vi "_Dequeue JKISMQ.vi"(8 "Error in":errorcluster caption="Error in (no error)", 9 "Dequeue Timeout(0ms)":i32, 10 "State(s) in (\"\")":string, 11 "JKISMQ in":T1) -> (0 "Error out":errorcluster, 2 "States Out":string, 3 "JKISMQ out":T1)   [LabVIEW 2014, in "JKI State Machine++.lvlib"]
uses:
  JKI State Machine++.lvlib
  _JKISMQ.ctl
  Typedef/_Cross JKISM State Data.ctl
  Typedef/_JKISM_MSG_TYPE.ctl
  Typedef/_Cross JKISM State Response.ctl
  Typedef/_JKISM_MODE.ctl
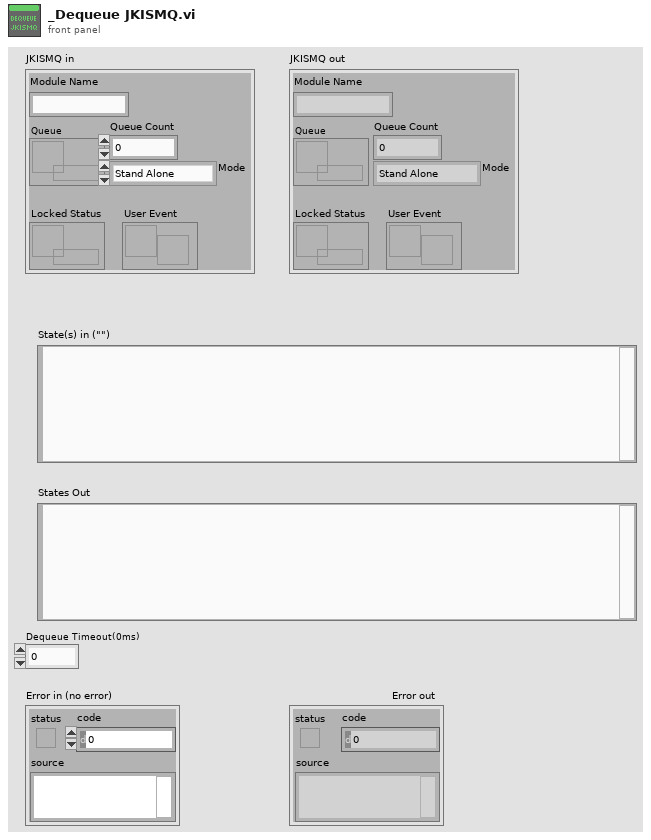
[diagram p1: front panel]
types:
  T1 = typedef "JKI State Machine++.lvlib/_JKISMQ.ctl" = cluster{"Module Name":string, "Queue":refnum<queue>, "Locked Status":refnum<data-value>, "Mode":T2, "User Event":refnum<user-event>, "Queue Count":i32}
  T2 = typedef "JKI State Machine++.lvlib/_JKISM_MODE.ctl" = enum16{"Stand Alone", "JKISM", "Action Worker"}
  T3 = typedef "JKI State Machine++.lvlib/_Cross JKISM State Data.ctl" = cluster{"Msg Type":T4, "state":string, "args":string, "source":string, "RespQ":refnum<queue>, "Pre-State":string, "Arg-State":string}
  T4 = typedef "JKI State Machine++.lvlib/_JKISM_MSG_TYPE.ctl" = enum16{"Sync Message(-@)", "Async Message(->)", "Async Response", "Broadcast(-><status>)", "Broadcast(-><interrupt>)"}
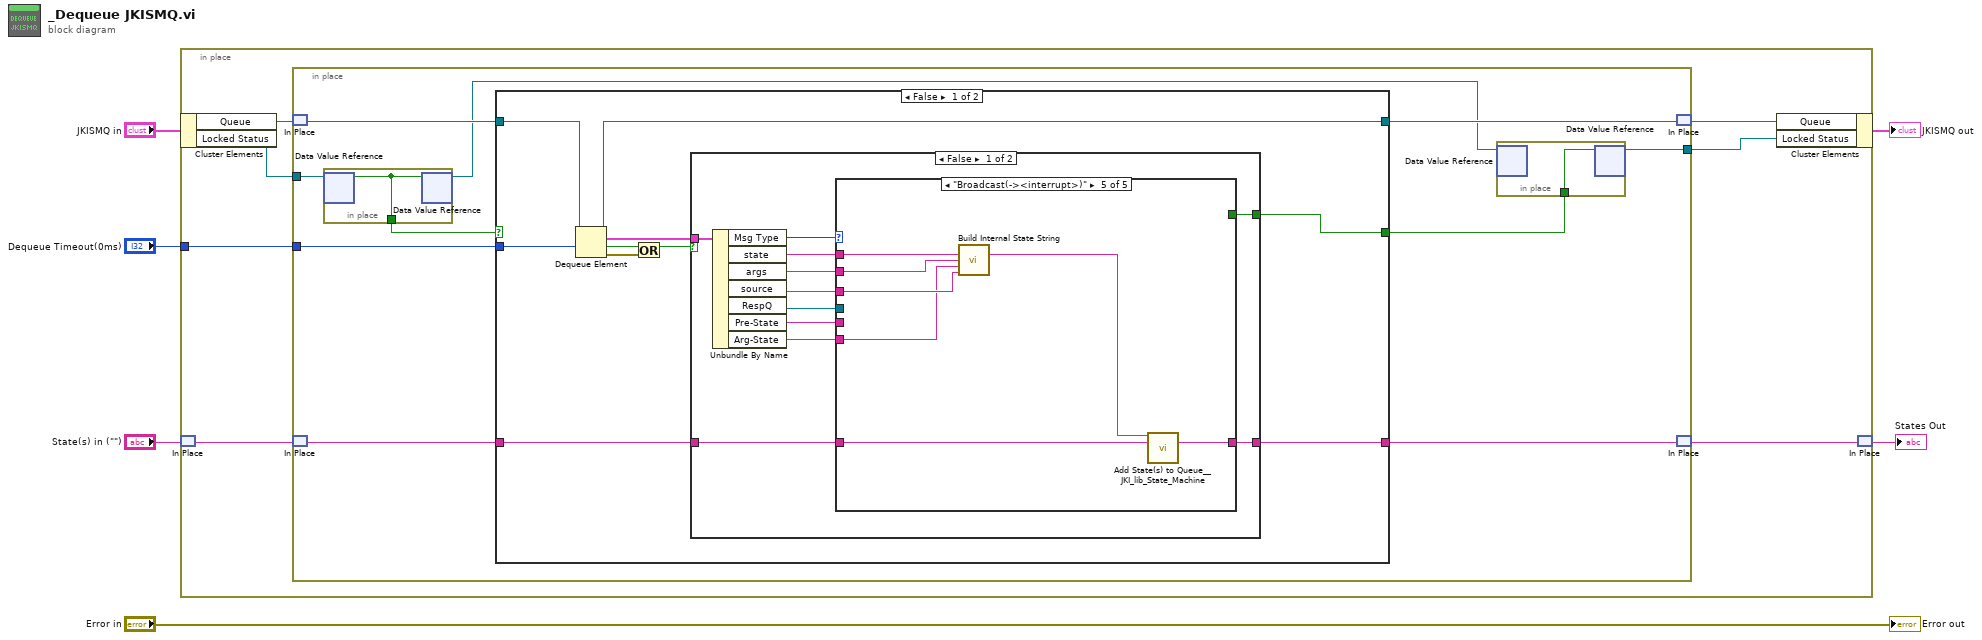
[diagram p0: block diagram]
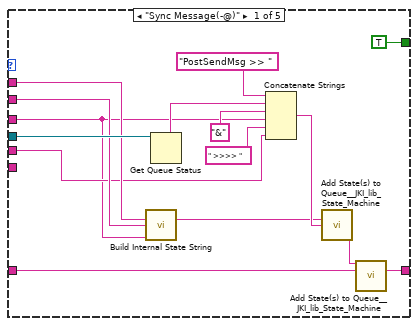
[diagram p2: hidden frame]
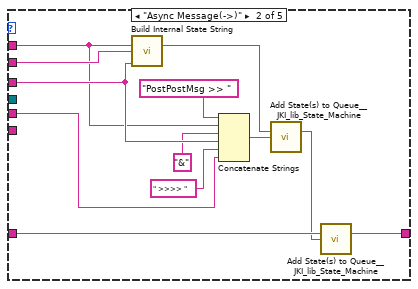
[diagram p3: hidden frame]
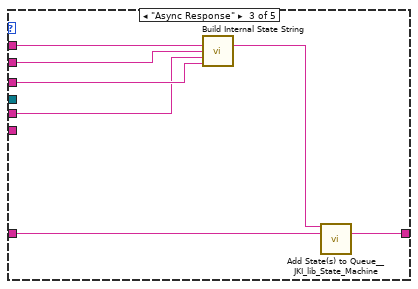
[diagram p4: hidden frame]
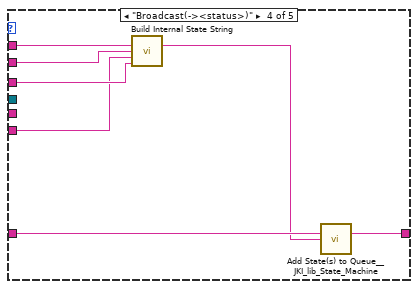
[diagram p5: hidden frame]
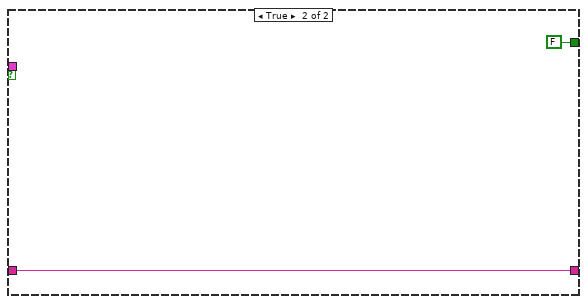
[diagram p6: hidden frame]
diagram:
  n1 = in-place "In Place Element Structure" {
    in-place-border: "Dequeue Timeout(0ms)" -> [w11]
    n2 = in-place-cluster #1("JKISMQ in") -> ("Queue"=w13:refnum<queue>, "Locked Status"=w8:refnum<data-value>)
    n3 = in-place-match #2("State(s) in (\"\")") -> (w10:string)
    n4 = in-place {
      in-place-border: w11 -> [w21]
      in-place-border: w8 -> [w18]
      in-place-border: [w15] -> w7
      n5 = in-place-match #3(w13) -> (w22:refnum<queue>)
      n6 = in-place-match #4(w10) -> (w20:string)
      n7 = in-place {
        in-place-border: [w25] -> w17
        n8 = in-place-dvr #5(w18) -> (w25:bool)  [unwired: 1 out]
        n9 = in-place-dvr #5(w25) -> (w16:refnum<data-value>)  [unwired: 1 out]
      }
      n10 = case shown="False" w17 {
        selector: w17 -> [_ w97]
        tunnel: [w34 w99] -> w23
        tunnel: w22 -> [w35 w99]
        tunnel: w21 -> [w33 _]
        tunnel: w20 -> [w31 w98]
        tunnel: [w30 w98] -> w19
        tunnel: [w29 w97] -> w14
        frame False {
          n11 = Dequeue Element(queue=w35, timeout in ms (-1)=w33) -> (queue out=w34:refnum<queue>, element=w32:T3, timed out?=w27:bool, error out=w26:errorcluster)  [unwired: 1 in]
          n12 = Or(x=w27, y=w26) -> (x .or. y?=w28:bool)
          n13 = case shown="False" w28 {
            tunnel: w31 -> [w46 w96]
            tunnel: [w45 w96] -> w30
            tunnel: w32 -> [w40 _]
            tunnel: [w39 FALSE] -> w29
            frame False {
              n14 = Unbundle By Name(w40) -> ("Msg Type"=w36:T4, "state"=w43:string, "args"=w42:string, "source"=w41:string, "RespQ"=w44:refnum<queue>, "Pre-State"=w38:string, "Arg-State"=w37:string)
              n15 = case shown="\"Broadcast(-><interrupt>)\"" w36 {
                tunnel: w46 -> [w61 w73 w80 w87 w94]
                tunnel: [w60 w72 w79 w86 w93] -> w45
                tunnel: w44 -> [w59 _ _ _ _]
                tunnel: w43 -> [w54 w69 w76 w83 w90]
                tunnel: w42 -> [w53 w71 w78 w85 w92]
                tunnel: w41 -> [w47 w70 w77 w84 w91]
                tunnel: [TRUE _ _ _ _] -> w39
                tunnel: w38 -> [w48 w68 w75 _ _]
                tunnel: w37 -> [_ _ _ w82 w89]
                frame "Sync Message(-@)" {
                  n16 = call "Build Internal State String.vi"("State"=w54, "Arguments (\"\")"=w53, "Source (\"\")"=w47) -> ("State with Arguments"=w55:string)  [unwired: 12 in]
                  n17 = Get Queue Status(queue=w59) -> (queue name=w52:string)  [unwired: 2 in, 7 out]
                  n18 = Concatenate Strings("PostSendMsg >> " ("State(s) at Back (\"\")"), w52, "&" ("string"), w47, " >>>> " ("string"), w48) -> (w56:string)
                  n19 = call <vilib>:"Add State(s) to Queue__JKI_lib_State_Machine.vi"("State(s) in (\"\")"=w55, "State(s) at Back (\"\")"=w56) -> ("States Out"=w58:string)  [unwired: 13 in]
                  n20 = call <vilib>:"Add State(s) to Queue__JKI_lib_State_Machine.vi"("State(s) in Front (\"\")"=w58, "State(s) in (\"\")"=w61) -> ("States Out"=w60:string)  [unwired: 13 in]
                }
                frame "Async Message(->)" {
                  n21 = call "Build Internal State String.vi"("State"=w69, "Arguments (\"\")"=w71, "Source (\"\")"=w70) -> ("State with Arguments"=w64:string)  [unwired: 12 in]
                  n22 = Concatenate Strings("PostPostMsg >> " ("State(s) at Back (\"\")"), w69, "&" ("string"), w70, " >>>> " ("string"), w68) -> (w63:string)
                  n23 = call <vilib>:"Add State(s) to Queue__JKI_lib_State_Machine.vi"("State(s) in (\"\")"=w64, "State(s) at Back (\"\")"=w63) -> ("States Out"=w67:string)  [unwired: 13 in]
                  n24 = call <vilib>:"Add State(s) to Queue__JKI_lib_State_Machine.vi"("State(s) in (\"\")"=w73, "State(s) at Back (\"\")"=w67) -> ("States Out"=w72:string)  [unwired: 13 in]
                }
                frame "Async Response" {
                  n25 = call "Build Internal State String.vi"("State"=w76, "Arguments (\"\")"=w78, "Arg-State (\"\")"=w75, "Source (\"\")"=w77) -> ("State with Arguments"=w74:string)  [unwired: 11 in]
                  n26 = call <vilib>:"Add State(s) to Queue__JKI_lib_State_Machine.vi"("State(s) in Front (\"\")"=w74, "State(s) in (\"\")"=w80) -> ("States Out"=w79:string)  [unwired: 13 in]
                }
                frame "Broadcast(-><status>)" {
                  n27 = call "Build Internal State String.vi"("State"=w83, "Arguments (\"\")"=w85, "Arg-State (\"\")"=w82, "Source (\"\")"=w84) -> ("State with Arguments"=w81:string)  [unwired: 11 in]
                  n28 = call <vilib>:"Add State(s) to Queue__JKI_lib_State_Machine.vi"("State(s) in (\"\")"=w87, "State(s) at Back (\"\")"=w81) -> ("States Out"=w86:string)  [unwired: 13 in]
                }
                frame "Broadcast(-><interrupt>)" {
                  n29 = call "Build Internal State String.vi"("State"=w90, "Arguments (\"\")"=w92, "Arg-State (\"\")"=w89, "Source (\"\")"=w91) -> ("State with Arguments"=w88:string)  [unwired: 11 in]
                  n30 = call <vilib>:"Add State(s) to Queue__JKI_lib_State_Machine.vi"("State(s) in Front (\"\")"=w88, "State(s) in (\"\")"=w94) -> ("States Out"=w93:string)  [unwired: 13 in]
                }
              }
            }
            frame True {
            }
          }
        }
        frame True {
        }
      }
      n31 = in-place {
        in-place-border: w14 -> [w24]
        n32 = in-place-dvr #6(w16) -> ()  [unwired: 2 out]
        n33 = in-place-dvr #6(w24) -> (w15:refnum<data-value>)  [unwired: 1 out]
      }
      n34 = in-place-match #3(w23) -> (w12:refnum<queue>)
      n35 = in-place-match #4(w19) -> (w9:string)
    }
    n36 = in-place-cluster #1("Queue"=w12, "Locked Status"=w7) -> (→"JKISMQ out":T1)
    n37 = in-place-match #2(w9) -> (→"States Out":string)
  }
  "Error out" <- "Error in"
